vi "Step Response - Air Heater.vi"() -> ()   [LabVIEW 2017]
uses:
  <vilib>/Simulation/Scripting/Companion Diagram/SimConfigNode/SimParams.ctl
  <vilib>/Simulation/Scripting/Companion Diagram/SimConfigNode/_simSolvers.ctl
  <vilib>/Simulation/Implementation/Shared/SIMSCR Execution Mode.ctl
  <vilib>/Simulation/Param Hierarchy/Typedefs/SIMPH Param Control Actions.ctl
  <vilib>/Simulation/Implementation/Shared/NILVSim_ParamChanged.vi
  <vilib>/Simulation/Implementation/Shared/NILVSIM_BeginStep.vi
  <vilib>/Simulation/Implementation/Shared/NILVSim_Manager.vi
  <vilib>/Utility/error.llb/Clear Errors.vi
  <vilib>/Simulation/Implementation/Shared/NILVSim_FinalizeModel.vi
  <vilib>/Simulation/Implementation/Shared/SIM Unbundle Sim Info.vi
  <vilib>/Simulation/Implementation/Shared/NILVSim_Initialize.vi
  <vilib>/Simulation/Utility/Implementation/NILVSim Get Time and IsAcceptedStep.vi
  <vilib>/Simulation/Implementation/Shared/SIMSH Read Queue.vi
  <vilib>/Simulation/Implementation/Shared/NILVSim_GetModelError.vi
  <vilib>/Simulation/Implementation/Shared/SIM Bundle Sim Info.vi
  <vilib>/Simulation/Implementation/XNodeFramework/SimXNode/SimX.xnode
  SubVIs/Air Heater Model.vi
  <vilib>/Simulation/Scripting/Companion Diagram/SimConfigNode/SimDog.xnode
  Air Heater Black Box Model.vi
  <vilib>/Simulation/Implementation/Shared/NI_SIM_Implementation.lvlib
panel:
  in  "Filename":path=path "data.lvm"
  in  "Enable Logging to File":bool caption="Enable"
  out "Control Chart":dbl(graph)=1.0
  out "Temperature Chart":dbl(graph)=28.561529046516153
  in  "Time Step [s]":dbl=0.1
  in  "Stop":bool
  in  "u":dbl(slide)=1.0 min=0.0 max=5.0 step=0.5 scale=0.0..5.0 scale format="%#.1g"
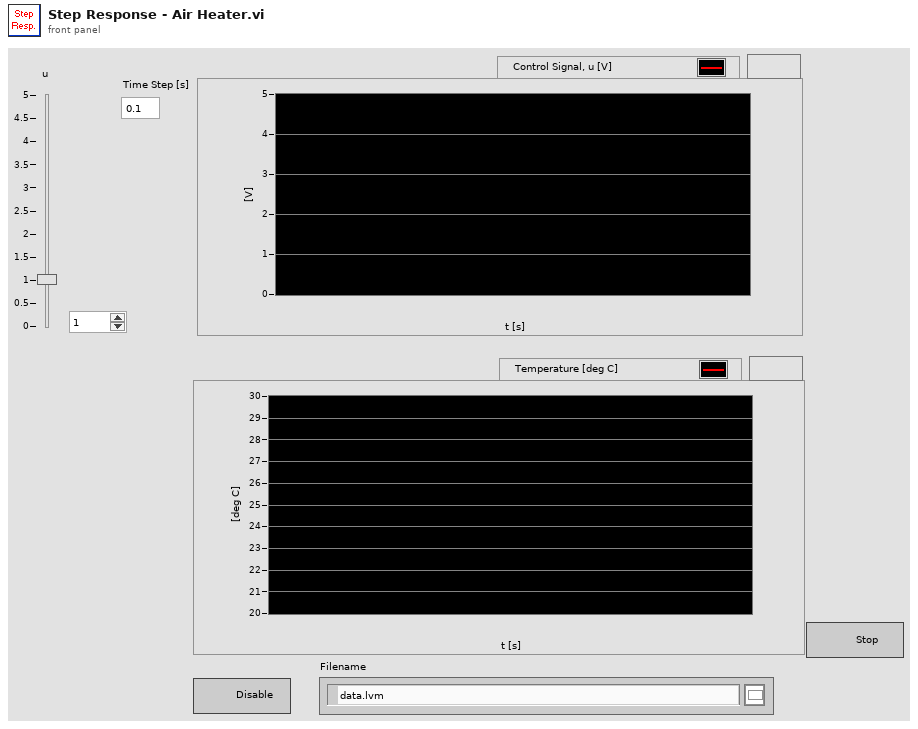
[diagram p1: front panel]
types:
  T1 = enum16{"Simulate to Completion", "Single Time-Step Simulation (Fixed Step Only)"}
  T2 = typedef "SIMSCR Execution Mode.ctl" = enum16{"Simulate to Completion", "Single Time-Step Simulation (Fixed Step Only)"}
  T3 = typedef "SIMPH Param Control Actions.ctl" = enum16{"get params", "set params"}
  T4 = cluster{"SIMSH Sim Time":dbl, "lower limit":dbl, "Integrator":cluster{"output":dbl}, "Multiplication":cluster{"Result":dbl}, "Summation":cluster{"Result":dbl}, "Multiplication 2":cluster{"Result":dbl}, "Transport Delay":cluster{"output":dbl}, "Summation 2":cluster{"Result":dbl}}
  T5 = typedef "SimParams.ctl" = cluster{"Initial Time (s)":dbl, "Final Time (s)":dbl, "Step Size (s)":dbl, "ODE Solver":T6, "Minimum Step Size (s)":dbl, "Maximum Step Size (s)":dbl, "Relative Tolerance":dbl, "Absolute Tolerance":dbl, "Software Timing":bool, "Initial Step Size (s)":dbl, "Automatic Fixed Step Size?":bool, "Automatic Discrete Step Size?":bool, "Discrete Step Size (s)":dbl, "Calculate using Time Step":bool, "Solver Wired?":bool, "Prev.Frm.Expected End":u64, "Prev.Frm.Actual End":u64, "Prev.Frm.Finished Late?":bool, "Prev.Iter.Expected End":u64, "Prev.Iter.Actual End":u64, "Prev.Iter.Finished Late?":bool, "Expected Iteration Start":u64, "Actual Iteration Start":u64, "Expected Frame Start":u64, "Actual Frame Start":u64, "Source Name":string, "Name":string, "Period":i64, "Deadline":i64, "Offset":i64, "Start":i64, "Priority":i32, "Timeout":i32, "Processor":i32, "Mode":enum32{"No Change", "Process missed periods, maintain original phase", "Discard missed periods, maintain original phase", "Process missed periods, ignore original phase", "Discard missed periods, ignore original phase"}, "Wakeup reason":enum32{"Normal", "Aborted", "Asynchronous wakeup", "Timing source error", "Timed loop error", "Timeout"}, "Error":errorcluster, "Source Type":string, "Secondary Source Type":string, "Global End Time":u64, "Global Start Time":u64, "Full Solver Reset":bool, "Execution Mode":T2, "Nan/Inf Check":bool, "Custom Solver Library":string, "Solver Is Variable":bool, "custom solver name":string, "Signal Collection Decimation":u32}
  T6 = typedef "_simSolvers.ctl" = enum16{"Runge-Kutta 1 (Euler)", "Runge-Kutta 2", "Runge-Kutta 3", "Runge-Kutta 4", "Runge-Kutta 23 (variable)", "Runge-Kutta 45 (variable)", "BDF (variable)", "Adams-Moulton (variable)", "Rosenbrock (variable)", "Discrete States Only", "SDIRK 4 (variable)", "Radau 5 (variable)", "Radau 9 (variable)", "Radau 13 (variable)", "Radau [Variable Order] (variable)", "Gear's Method (variable)", "Linearizer", "State Query", "Trim Eval", "Custom Solver"}
  T7 = cluster{"SIMSH Sim Time":dbl, "Select":cluster{"s? t:f":dbl}, "Linear Scaling with Points.vi":cluster{"y":dbl}, "Summation 3":cluster{"Result":dbl}, "Square Root":cluster{"sqrt(x)":dbl}, "Gaussian White Noise PtByPt.vi":cluster{"Gaussian white noise":dbl}, "Integrator":cluster{"output":dbl}, "Multiplication":cluster{"Result":dbl}, "Summation":cluster{"Result":dbl}, "Multiplication 2":cluster{"Result":dbl}, "Transport Delay":cluster{"output":dbl}, "Summation 2":cluster{"Result":dbl}}
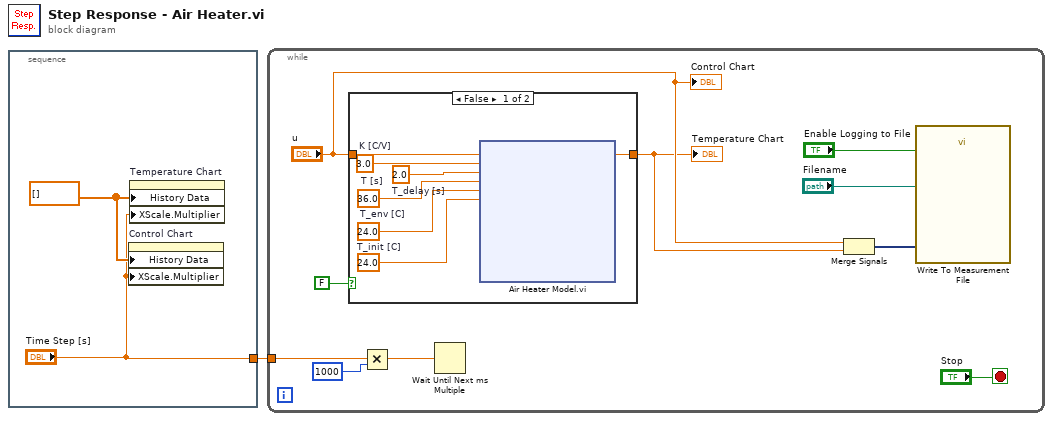
[diagram p0: block diagram]
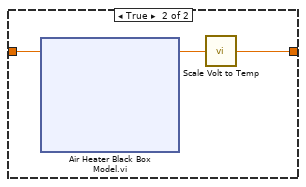
[diagram p2: hidden frame]
diagram:
  n1 = stacked-sequence {
    tunnel: ["Time Step [s]"] -> w1
    frame #0 {
      w3 = dbl[] [] ("History Data")
      n2 = property on="Control Chart" class="WFChart (strict)"("History Data"=w3, "XScale.Multiplier"="Time Step [s]") -> ()  [unwired: 2 in, 2 out]
      n3 = property on="Temperature Chart" class="WFChart (strict)"("History Data"=w3, "XScale.Multiplier"="Time Step [s]") -> ()  [unwired: 2 in, 2 out]
    }
  }
  n4 = while {
    tunnel: w1 -> [w12]
    stop <- "Stop" stop-if-true
    n5 = case shown="False" FALSE {
      tunnel: "u" -> [w19 w295]
      tunnel: [w20 w293] -> w7
      frame False {
        w14 = 24.0  # T_init [C]
        w15 = 24.0  # T_env [C]
        w16 = 36.0  # T [s]
        w17 = 2.0  # T_delay [s]
        w18 = 3.0  # K [C/V]
        n6 = xnode "Air Heater Model.vi"("u [V]"=w19, "K [C/V]"=w18, "T_delay [s]"=w17, "T [s]"=w16, "T_env [C]"=w15, "T_init [C]"=w14) -> ("Tout [C]"=w20:dbl)  [unwired: 2 in, 14 out]
      }
      frame True {
        n7 = xnode "Air Heater Black Box Model.vi"("Control Signal [0-5V]"=w295) -> ("Tout [1-5V]"=w294:dbl)  [unwired: 2 in, 1 out]
        n8 = call "Scale Volt to Temp.vi"("Input Value (V)"=w294) -> ("Output Value (degC)"=w293:dbl)
      }
    }
    "Temperature Chart" <- w7
    n9 = Multiply(x=w12, y=1000) -> (x*y=w10:dbl)
    n10 = Wait Until Next ms Multiple(millisecond multiple=w10) -> ()  [unwired: 1 out]
    n11 = Merge Signals("u", w7) -> (w6:dynamicdata)
    n12 = call "Write To Measurement File"("Signals"=w6, "Enable"="Enable Logging to File", "Filename"="Filename") -> ()  [unwired: 14 in, 3 out]
    "Control Chart" <- "u"
  }
